vi "Ctor.vi"(8 "error in (no error)":errorcluster, 11 "AppDetailPanel in":refnum<class "AppDetailPanel.lvclass">) -> (0 "error out":errorcluster, 3 "AppDetailPanel out":refnum<class "AppDetailPanel.lvclass">)   [LabVIEW 2020, in "PicoG-App.lvlib" / "AppDetailPanel.lvclass"]
uses:
  AppDetailPanel.lvclass
  ViaApp/ViaApp.lvclass
  Ref Data.ctl
  <vilib>/IlluminatedG/IG OOPanel/OOPanel/Panel/Panel.lvclass
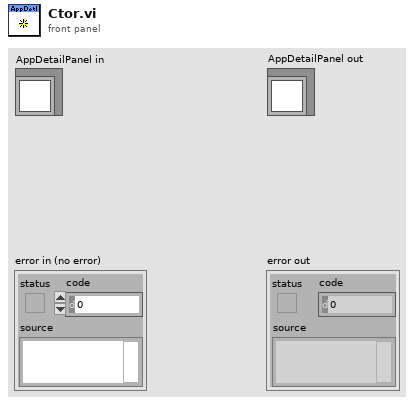
[diagram p1: front panel]
types:
  T1 = typedef "PicoG-App.lvlib/AppDetailPanel.lvclass/Ref Data.ctl" = cluster{"App":refnum<class "ViaApp.lvclass">}
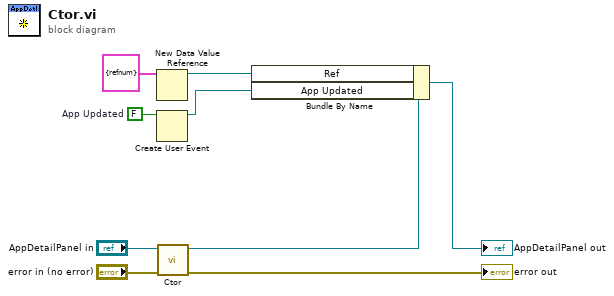
[diagram p0: block diagram]
diagram:
  w2 = FALSE  # App Updated
  n1 = New Data Value Reference(data value=T1 {"App"=refnum} ("Ref Data")) -> (data value reference=w7:refnum<data-value>)  [unwired: 1 in, 1 out]
  n2 = Create User Event(user event datatype=w2) -> (user event=w1:refnum<user-event>)  [unwired: 1 in, 1 out]
  n3 = call-parent "Ctor.vi"("error in (no error)"="error in (no error)", "Panel in"="AppDetailPanel in") -> ("error out"=→"error out":errorcluster, "Panel out"=w5:refnum<class "AppDetailPanel.lvclass">)  [unwired: 8 in]
  n4 = Bundle By Name(cluster=w5, "Ref"=w7, "App Updated"=w1) -> (→"AppDetailPanel out":refnum<class "AppDetailPanel.lvclass">)
